vi "Do.vi"(8 "error in (no error)":errorcluster, 10 "Actor in":refnum<class "Actor.lvclass">, 11 "ScanDone Msg":refnum<class "ScanDone Msg.lvclass">) -> (0 "error out":errorcluster, 2 "Actor out":refnum<class "Actor.lvclass">)   [LabVIEW 2023, in "ControllerComm.lvlib" / "ScanDone Msg.lvclass"]
doc: "This VI delivers the message to the actor by calling the appropriate method(s) on the actor."
uses:
  ScanDone Msg.lvclass
  <vilib>/ActorFramework/Actor/Actor.lvclass
  Controller Comm/CommToUI.lvclass
  9ef47adc-f318-494c-9b8b-6df3216d6863.vi
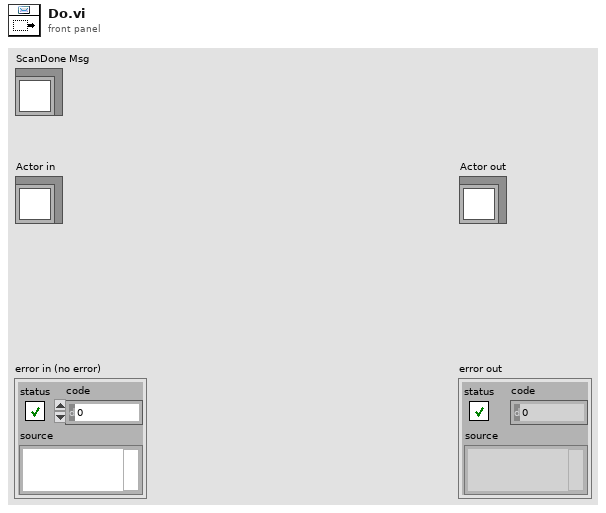
[diagram p1: front panel]
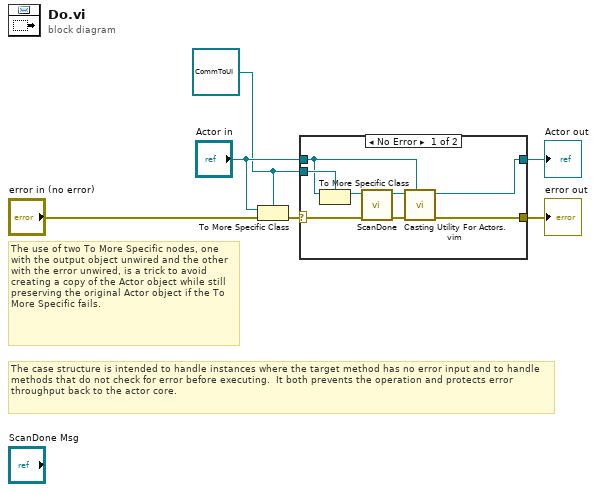
[diagram p0: block diagram]
diagram:
  w1 = refnum<class "CommToUI.lvclass"> refnum ("ControllerComm.lvlib:CommToUI.lvclass")
  # "The use of two To More Specific nodes, one with the output object unwired and the other with the error unwired, is a trick to avoid creating a copy of the Actor object while still preserving the original Actor object if the To More Specific fails."
  # "The case structure is intended to handle instances where the target method has no error input and to handle methods that do not check for error before executing.  It both prevents the operation and protects error throughput back to the actor core."
  n1 = To More Specific Class(target class=w1, reference="Actor in", error in="error in (no error)") -> (error out=w5:errorcluster)  [unwired: 1 out]
  n2 = case shown="No Error" w5 {
    selector: w5 -> [w8 w16]
    tunnel: [w11 w16] -> w4
    tunnel: [w12 w15] -> w3
    tunnel: "Actor in" -> [w13 w15]
    tunnel: w1 -> [w14 _]
    frame No Error {
      n3 = To More Specific Class(target class=w14, reference=w13) -> (specific class reference=w10:refnum<class "CommToUI.lvclass">)  [unwired: 1 in, 1 out]
      n4 = call-dynamic "ScanDone.vi"("error in (no error)"=w8, "ControllerComm.lvlib:CommToUI.lvclass"=w10) -> ("error out"=w7:errorcluster, "ControllerComm.lvlib:CommToUI.lvclass"=w9:refnum<class "CommToUI.lvclass">)  [unwired: 8 in]
      n5 = call "Casting Utility For Actors.vim"("type"=w13, "error in (no error)"=w7, "Actor in"=w9) -> ("error out"=w11:errorcluster, "Actor out"=w12:refnum<class "Actor.lvclass">)  [unwired: 7 in]
    }
    frame Error {
      # "If type check fails, pass the original object out again."
    }
  }
  "error out" <- w4
  "Actor out" <- w3
